vi "例9.6 播放一首音乐.vi"() -> ()   [LabVIEW 2012]
doc: "本VI将直接播放声音文件并输出至扬声器。通过Play Sound File.vi打开文件并马上开始异步播放（相对于Sound File to Sound Output.vi范例中显示的方法）。"
panel:
  out "音乐波形":waveform(dbl)[](graph)
  in  "path":path caption="路径"
  in  "Device ID":u32 caption="设备ID" format="%.0x"
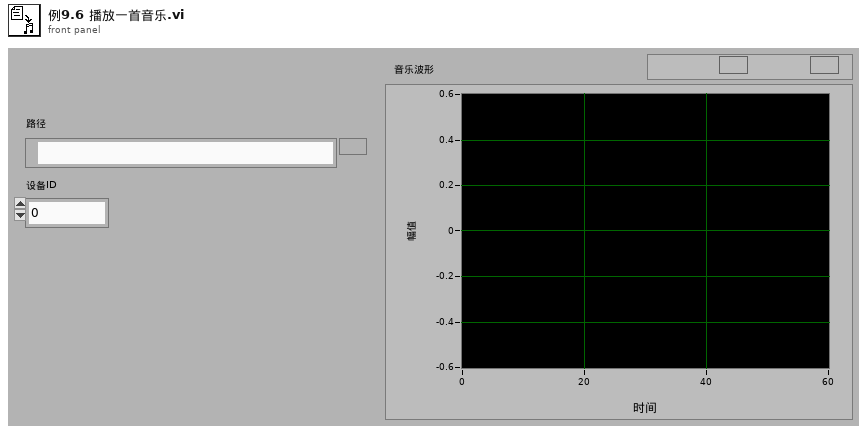
[diagram p1: front panel]
types:
  T1 = typedef "Sound Output Task ID.ctl" = u32
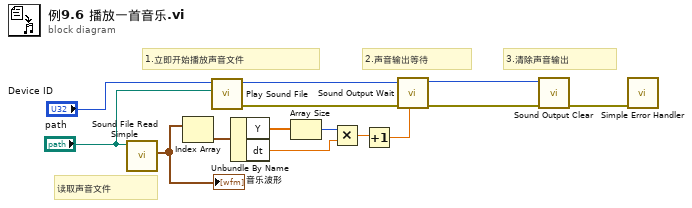
[diagram p0: block diagram]
diagram:
  # "2.声音输出等待"
  # "3.清除声音输出"
  # "1.立即开始播放声音文件"
  # "读取声音文件"
  n1 = call <vilib>:"Sound File Read Simple.vi"("path"="path") -> ("data"=w10:waveform(dbl)[])  [unwired: 7 in, 3 out]
  "音乐波形" <- w10
  n2 = Index Array(array=w10) -> (element=w9:waveform(dbl))  [unwired: 1 in]
  n3 = call <vilib>:"Play Sound File.vi"("path"="path", "device ID"="Device ID") -> ("error out"=w12:errorcluster, "task ID"=w13:T1)  [unwired: 8 in]
  n4 = Unbundle By Name(w9) -> ("Y"=w8:dbl[], "dt"=w2:dbl)
  n5 = Array Size(array=w8) -> (size(s)=w4:i32)
  n6 = Multiply(x=w4, y=w2) -> (x*y=w7:dbl)
  n7 = Increment(x=w7) -> (x+1=w3:dbl)
  n8 = call <vilib>:"Sound Output Wait.vi"("timeout (sec)"=w3, "error in (no error)"=w12, "task ID"=w13) -> ("error out"=w5:errorcluster, "task ID out"=w6:T1)  [unwired: 7 in]
  n9 = call <vilib>:"Sound Output Clear.vi"("error in (no error)"=w5, "task ID"=w6) -> ("error out"=w1:errorcluster)  [unwired: 9 in]
  n10 = call <vilib>:"Simple Error Handler.vi"("error in (no error)"=w1) -> ()  [unwired: 4 in, 5 out]
